vi "updateProductDataInProductTable.vi"(8 "error in":errorcluster, 11 "dataReadingToUpdate":T1) -> (0 "error out":errorcluster, 3 "dataUpdate":T1)   [LabVIEW 2014]
uses:
  <vilib>/addons/database/NI_Database_API.lvlib
  <vilib>/addons/database/Connection.llb/DB Tools Open Connec (String).vi
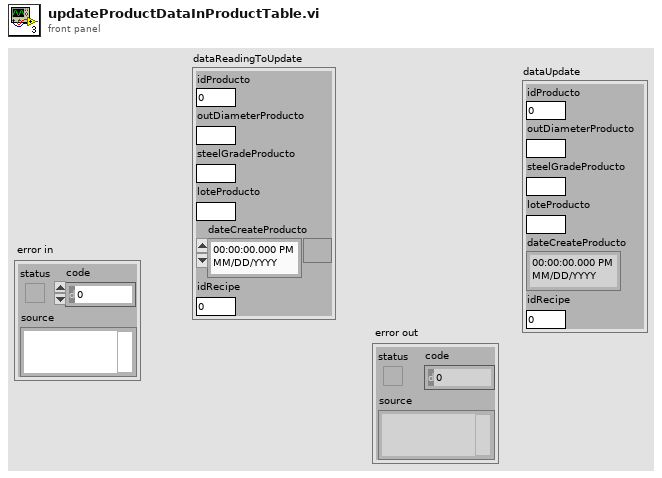
[diagram p1: front panel]
types:
  T1 = cluster{"idProducto":dbl, "outDiameterProducto":string, "steelGradeProducto":string, "loteProducto":string, "dateCreateProducto":timestamp, "idRecipe":dbl}
  T2 = typedef "NI_Database_API.lvlib/Conn ObjectReference.ctl" = refnum<k1>
  T3 = typedef "NI_Database_API.lvlib/DB Tools DataTypes.ctl" = enum16{"String", "Long (I32)", "Single (SGL)", "Double (DBL)", "Date/Time", "Binary"}
  T4 = cluster{"name":string, "database data type":T3, "defined size":i32}[]
  T5 = cluster{cluster{string, string, string, string, string}, string[]}
  T6 = cluster{cluster{string, string, string}, string[]}
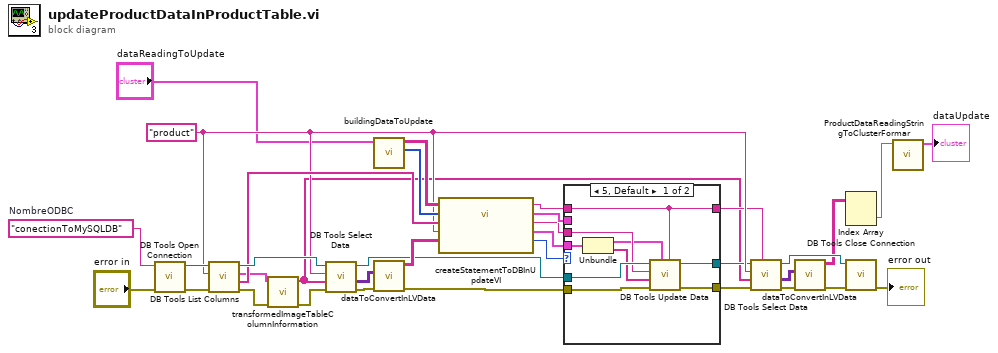
[diagram p0: block diagram]
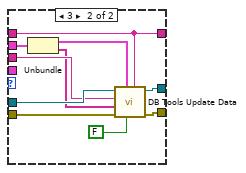
[diagram p2: hidden frame]
diagram:
  w15 = "product" ("tableName")
  w35 = "conectionToMySQLDB"  # NombreODBC
  n1 = call-poly <vilib>:"DB Tools Open Connection.vi"("error in (no error)"="error in", "connection information"=w35) -> ("error out"=w32:errorcluster, "connection reference"=w33:T2)  [unwired: 6 in]
  n2 = call <vilib>:"DB Tools List Columns.vi"("error in (no error)"=w32, "table"=w15, "connection reference"=w33) -> ("error out"=w5:errorcluster, "columns"=w21:string[], "column information"=w6:T4, "connection reference out"=w31:T2)  [unwired: 1 in]
  n3 = call "transformedImageTableColumnInformation.vi"("error in"=w5, "columnInformationReading"=w6) -> ("error out"=w4:errorcluster, "columnInformationReadingTransformed"=w3:string[])  [unwired: 8 in]
  n4 = call <vilib>:"DB Tools Select Data.vi"("error in (no error)"=w4, "columns"=w3, "table"=w15, "connection reference"=w31) -> ("error out"=w30:errorcluster, "data"=w29:variant[][], "connection reference out"=w19:T2)  [unwired: 2 in]
  n5 = call "buildingDataToUpdate.vi"("dataReadingToUpdate"="dataReadingToUpdate") -> ("RawIndexToModifyOut"=w17:i32[], "ItemNamesOut"=w18:string[][])  [unwired: 9 in]
  n6 = call "dataToConvertInLVData.vi"("error in"=w30, "dataReadingIn"=w29) -> ("error out"=w20:errorcluster, "dataReadingOut"=w22:string[][])  [unwired: 8 in]
  n7 = call "createStatementToDBInUpdateVI.vi"("DataReadingInTableBeforeToUpdate"=w22, "Nombre Tabla"=w15, "ColumnName"=w21, "RawIndexToModify"=w17, "ItemNames"=w18) -> ("DataToModify5"=w26:T5, "TableNameToModify"=w25:string, "DataToModify3"=w27:T6, "statementSQL"=w28:string, "NumberOfFields"=w24:i32)  [unwired: 2 in]
  n8 = case shown="5, Default" w24 {
    tunnel: w19 -> [w41 w54]
    tunnel: w20 -> [w42 w53]
    tunnel: [w43 w52] -> w14
    tunnel: [w44 w51] -> w16
    tunnel: w25 -> [w40 w50]
    tunnel: w28 -> [w36 w45]
    tunnel: w27 -> [_ w48]
    tunnel: w26 -> [w39 _]
    tunnel: [w36 w45] -> w13
    frame 5, Default {
      n9 = Unbundle(w39) -> (w38:cluster{string, string, string, string, string}, w37:string[])
      n10 = call <vilib>:"DB Tools Update Data.vi"("condition"=w36, "data"=w38, "error in (no error)"=w42, "columns"=w37, "table"=w40, "connection reference"=w41) -> ("error out"=w44:errorcluster, "connection reference out"=w43:T2)  [unwired: 4 in]
    }
    frame 3 {
      n11 = Unbundle(w48) -> (w47:cluster{string, string, string}, w46:string[])
      n12 = call <vilib>:"DB Tools Update Data.vi"("condition"=w45, "flatten cluster? (F)"=FALSE, "data"=w47, "error in (no error)"=w53, "columns"=w46, "table"=w50, "connection reference"=w54) -> ("error out"=w51:errorcluster, "connection reference out"=w52:T2)  [unwired: 3 in]
    }
  }
  n13 = call <vilib>:"DB Tools Select Data.vi"("condition"=w13, "error in (no error)"=w16, "columns"=w3, "table"=w15, "connection reference"=w14) -> ("error out"=w9:errorcluster, "data"=w10:variant[][], "connection reference out"=w12:T2)  [unwired: 1 in]
  n14 = call "dataToConvertInLVData.vi"("error in"=w9, "dataReadingIn"=w10) -> ("error out"=w8:errorcluster, "dataReadingOut"=w11:string[][])  [unwired: 8 in]
  n15 = Index Array(array=w11) -> (element=w7:string[])  [unwired: 2 in]
  n16 = call <vilib>:"DB Tools Close Connection.vi"("error in (no error)"=w8, "connection reference"=w12) -> ("error out"=→"error out":errorcluster)  [unwired: 5 in]
  n17 = call "ProductDataReadingStringToClusterFormar.vi"("StringFormat"=w7) -> ("ClusterFormat"=→"dataUpdate":T1)  [unwired: 10 in]
